vi "Model - Init.vi"(8 "error in (no error)":errorcluster) -> (0 "error out":errorcluster, 3 "View Model":T1)   [LabVIEW 2017]
doc: "Initialize View Model by actual values of User Event and DVR"
uses:
  Controls/View Model.ctl
  Error Handler/Controls/Error Model.ctl
  Error Handler/Controls/Error EventData.ctl
  Error Handler/Controls/Error Type.ctl
  Elevator Controller/Controls/Elevator Model.ctl
  Elevator Controller/Controls/Elevator Overhead.ctl
  Elevator Controller/Controls/Elevator States.ctl
  Elevator Controller/Controls/Elevator Location.ctl
  Elevator Controller/Controls/Elevator Command Event.ctl
  Elevator Controller/Controls/Elevator Commands.ctl
  Configuration/Controls/Configuration Model.ctl
  Configuration/Controls/Configuration Data.ctl
  Controls/Shared Model.ctl
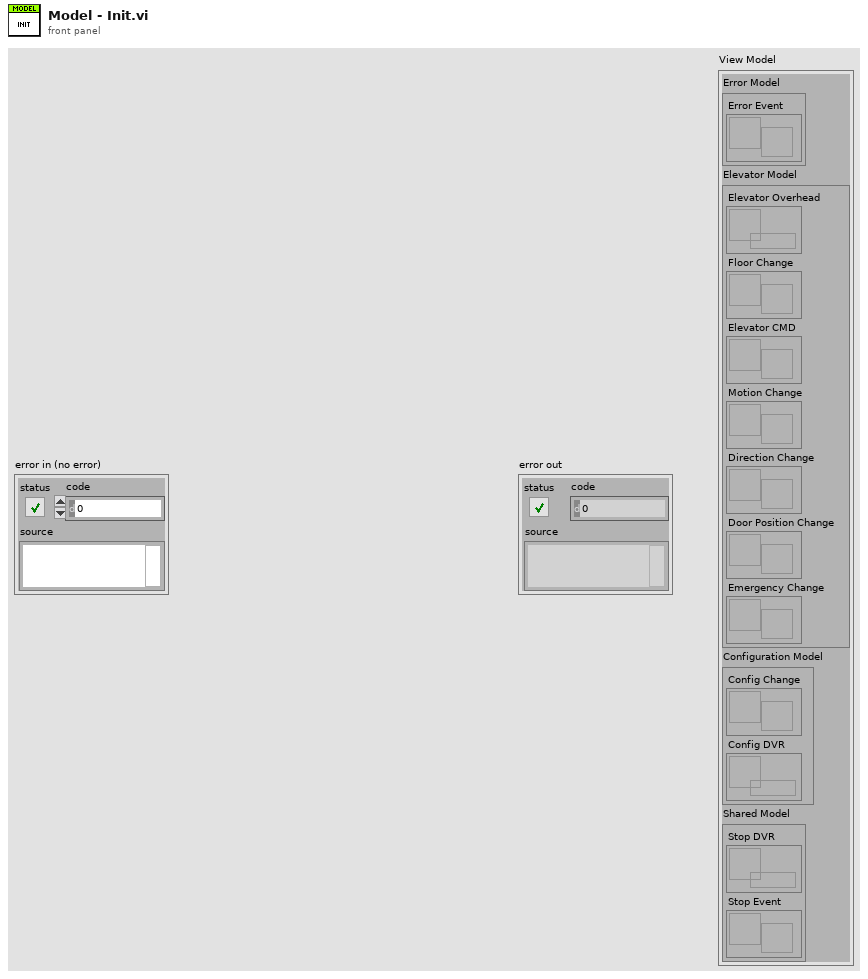
[diagram p1: front panel]
types:
  T1 = typedef "View Model.ctl" = cluster{"Error Model":T2, "Elevator Model":T3, "Configuration Model":T4, "Shared Model":T5}
  T2 = typedef "Error Model.ctl" = cluster{"Error Event":refnum<user-event>}
  T3 = typedef "Elevator Model.ctl" = cluster{"Elevator Overhead":refnum<data-value>, "Floor Change":refnum<user-event>, "Elevator CMD":refnum<user-event>, "Motion Change":refnum<user-event>, "Direction Change":refnum<user-event>, "Door Position Change":refnum<user-event>, "Emergency Change":refnum<user-event>}
  T4 = typedef "Configuration Model.ctl" = cluster{"Config Change":refnum<user-event>, "Config DVR":refnum<data-value>}
  T5 = typedef "Shared Model.ctl" = cluster{"Stop DVR":refnum<data-value>, "Stop Event":refnum<user-event>}
  T6 = typedef "Elevator Location.ctl" = enum16{"1st Floor", "2nd Floor", "3rd Floor", "4th Floor"}
  T7 = typedef "Elevator Command Event.ctl" = cluster{"Elevator Commands":T8, "Variant":variant}
  T8 = typedef "Elevator Commands.ctl" = enum16{"Go Up", "Go Down", "Go to Floor", "Emergency", "Open Doors", "Close Doors"}
  T9 = typedef "Elevator Overhead.ctl" = cluster{"Elevator State":T10, "Next Elevator State":T10, "In Motion?":bool, "Direction":bool, "Door Movement":bool, "Door Position":bool, "Timer":dbl, "Elapsed Time":dbl}
  T10 = typedef "Elevator States.ctl" = enum16{"Idle", "Init", "Open Doors", "Close Doors", "Start Move", "Move", "Finish Move", "Analysis", "Emergency"}
  T11 = typedef "Error EventData.ctl" = cluster{"Error Type":T12, "error in (no error)":errorcluster}
  T12 = typedef "Error Type.ctl" = enum16{"Console Error", "Sensor Interface IO Error", "Process Step Error"}
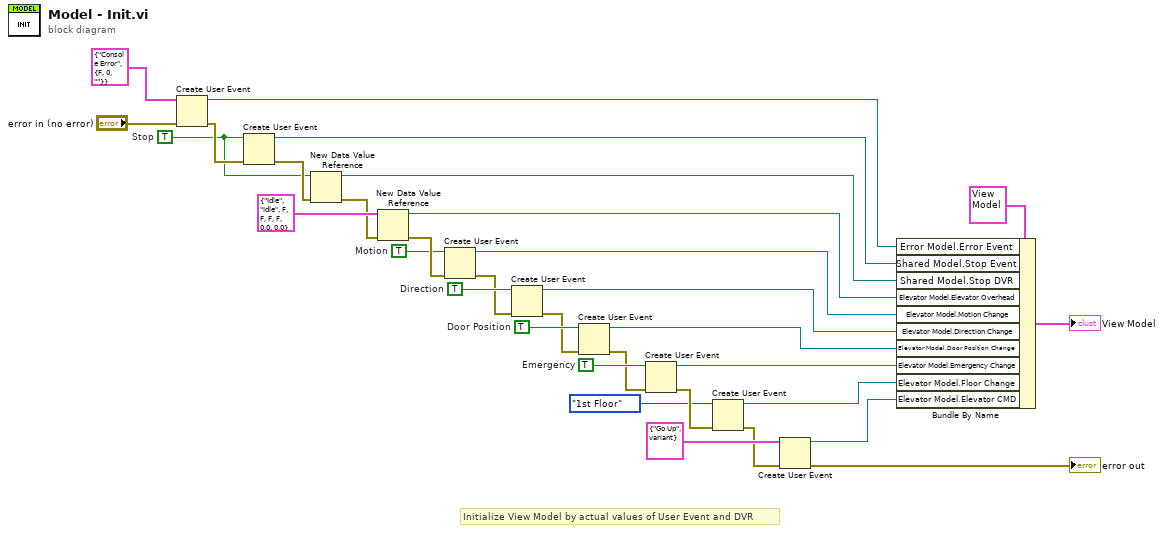
[diagram p0: block diagram]
diagram:
  w19 = TRUE  # Emergency
  w21 = TRUE  # Door Position
  w23 = TRUE  # Direction
  w24 = TRUE  # Motion
  w28 = TRUE  # Stop
  # "Initialize View Model by actual values of User Event and DVR"
  n1 = Create User Event(user event datatype=T11 {"Error Type"=enum."Console Error", "error in (no error)"={"status"=FALSE, "code"=0, "source"=""}} ("Error Event Data"), error in="error in (no error)") -> (user event=w12:refnum<user-event>, error out=w30:errorcluster)
  n2 = Create User Event(user event datatype=w28, error in=w30) -> (user event=w8:refnum<user-event>, error out=w29:errorcluster)
  n3 = New Data Value Reference(data value=w28, error in=w29) -> (data value reference=w7:refnum<data-value>, error out=w26:errorcluster)
  n4 = New Data Value Reference(data value=T9 {"Elevator State"=enum."Idle", "Next Elevator State"=enum."Idle", "In Motion?"=FALSE, "Direction"=FALSE, "Door Movement"=FALSE, "Door Position"=FALSE, "Timer"=0.0, "Elapsed Time"=0.0} ("Elevator Overhead"), error in=w26) -> (data value reference=w6:refnum<data-value>, error out=w25:errorcluster)
  n5 = Create User Event(user event datatype=w24, error in=w25) -> (user event=w5:refnum<user-event>, error out=w22:errorcluster)
  n6 = Create User Event(user event datatype=w23, error in=w22) -> (user event=w4:refnum<user-event>, error out=w20:errorcluster)
  n7 = Create User Event(user event datatype=w21, error in=w20) -> (user event=w3:refnum<user-event>, error out=w18:errorcluster)
  n8 = Create User Event(user event datatype=w19, error in=w18) -> (user event=w2:refnum<user-event>, error out=w17:errorcluster)
  n9 = Create User Event(user event datatype=Elevator_Location."1st Floor" ("Elevator Location"), error in=w17) -> (user event=w1:refnum<user-event>, error out=w14:errorcluster)
  n10 = Create User Event(user event datatype=T7 {"Elevator Commands"=enum."Go Up", "Variant"=variant} ("Elevator CMD Event"), error in=w14) -> (user event=w13:refnum<user-event>, error out=→"error out":errorcluster)
  n11 = Bundle By Name(cluster=T1 {"Error Model"={"Error Event"=refnum}, "Elevator Model"={"Elevator Overhead"=refnum, "Floor Change"=refnum, "Elevator CMD"=refnum, "Motion Change"=refnum, "Direction Change"=refnum, "Door Position Change"=refnum, "Emergency Change"=refnum}, "Configuration Model"={"Config Change"=refnum, "Config DVR"=refnum}, "Shared Model"={"Stop DVR"=refnum, "Stop Event"=refnum}} ("View Model"), "Error Model.Error Event"=w12, "Shared Model.Stop Event"=w8, "Shared Model.Stop DVR"=w7, "Elevator Model.Elevator Overhead"=w6, "Elevator Model.Motion Change"=w5, "Elevator Model.Direction Change"=w4, "Elevator Model.Door Position Change"=w3, "Elevator Model.Emergency Change"=w2, "Elevator Model.Floor Change"=w1, "Elevator Model.Elevator CMD"=w13) -> (→"View Model":T1)
